vi "Close.vi"(8 "error in (no error)":errorcluster, 11 ".NET Refnum in":refnum<k24>) -> (0 "error out":errorcluster)   [LabVIEW 2021]
uses:
  C:/Program Files/Thorlabs/Scientific Imaging/ThorCam/uc480DotNet.dll
  Program Files/Thorlabs/Scientific Imaging/ThorCam/uc480DotNet.dll
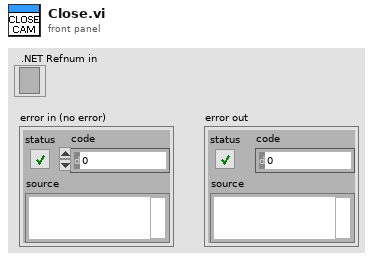
[diagram p1: front panel]
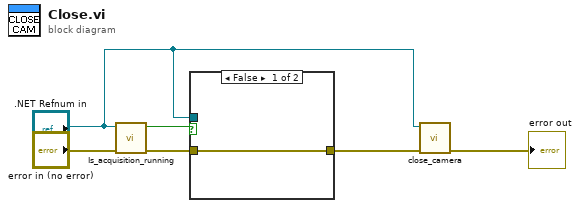
[diagram p0: block diagram]
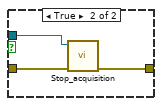
[diagram p2: hidden frame]
diagram:
  n1 = call "Is_acquisition_running.vi"("error in (no error)"="error in (no error)", "uc480.Camera"=".NET Refnum in") -> ("error out"=w1:errorcluster, "bValue"=w4:bool)  [unwired: 8 in]
  n2 = case shown="False" w4 {
    tunnel: w1 -> [w7 w10]
    tunnel: ".NET Refnum in" -> [_ w9]
    tunnel: [w7 w8] -> w2
    frame False {
    }
    frame True {
      n3 = call "Stop_acquisition.vi"("error in (no error)"=w10, "uc480.Camera"=w9) -> ("error out"=w8:errorcluster)  [unwired: 8 in, 1 out]
    }
  }
  n4 = call "close_camera.vi"("error in (no error)"=w2, "uc480.Camera"=".NET Refnum in") -> ("error out"=→"error out":errorcluster)  [unwired: 8 in, 1 out]
